vi "Assert Not Count.vi"(5 "Expected":i32, 7 "Message (\"\")":string, 8 "error in (no error)":errorcluster, 10 "Haystack":variant) -> (0 "error out":errorcluster)   [LabVIEW 2017, in "Assertion.lvlib"]
doc: "Asserts the number of elements in an array, set or map. Does nothing if an error occurred before this node runs. Returns an error if the assertion failed. Optionally adds a message to the error message if the assertion failed."
uses:
  Assertion.lvlib
  Constraint/LogicalNot/LogicalNot.lvclass
  Constraint/Count/Count.lvclass
  C:/Users/de200256/Code/logmanoriginal/lvunit/Constraint/Constraint/Constraint.lvclass
  Constraint/UnaryOperator/UnaryOperator.lvclass
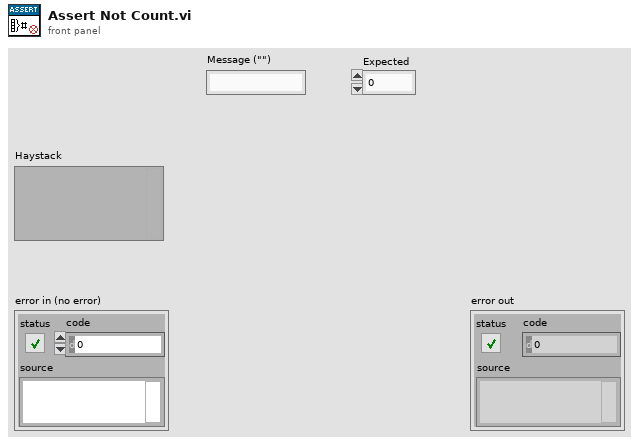
[diagram p1: front panel]
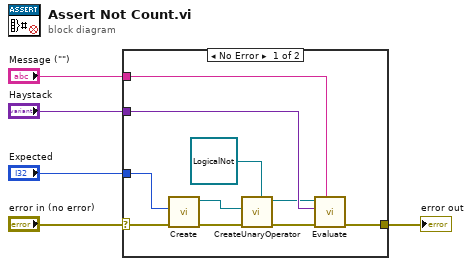
[diagram p0: block diagram]
diagram:
  n1 = case shown="No Error" "error in (no error)" {
    selector: "error in (no error)" -> [w10 w16]
    tunnel: [w15 w16] -> w5
    tunnel: "Haystack" -> [w14 _]
    tunnel: "Message (\"\")" -> [w13 _]
    tunnel: "Expected" -> [w12 _]
    frame No Error {
      n2 = call "Create.vi"("error in (no error)"=w10, "Expected"=w12) -> ("error out"=w11:errorcluster, "Count"=w7:refnum<class "Count.lvclass">)  [unwired: 8 in]
      n3 = call-dynamic "CreateUnaryOperator.vi"("UnaryOperator In"=refnum<class "LogicalNot.lvclass"> refnum ("Constraint.lvlib:LogicalNot.lvclass"), "error in (no error)"=w11, "Constraint"=w7) -> ("error out"=w9:errorcluster, "UnaryOperator"=w8:refnum<class "UnaryOperator.lvclass">)  [unwired: 7 in]
      n4 = call-dynamic "Evaluate.vi"("Message (\"\")"=w13, "error in (no error)"=w9, "Actual"=w14, "Constraint in"=w8) -> ("error out"=w15:errorcluster)  [unwired: 6 in, 1 out]
    }
    frame Error {
    }
  }
  "error out" <- w5
